vi "Problem 20 - Factorial digit sum.vi"() -> ()   [LabVIEW 2021, in "Project Euler.lvlib"]
uses:
  Project Euler.lvlib
  Utilities/Named Timers/Named Timers.lvlib
  Utilities/Numeric Utilities/Numeric Utilities.lvlib
panel:
  out "Answer = sum of digits of 100!":i32
  out "100!":string
  out "Total execution time (ms)":u32
  # "Input\nInputs to the VI"
  # "Development\nControls or indicators that are useful for development or testing, but which are not outputs of the VI."
  # "Output\nOutputs of the VI"
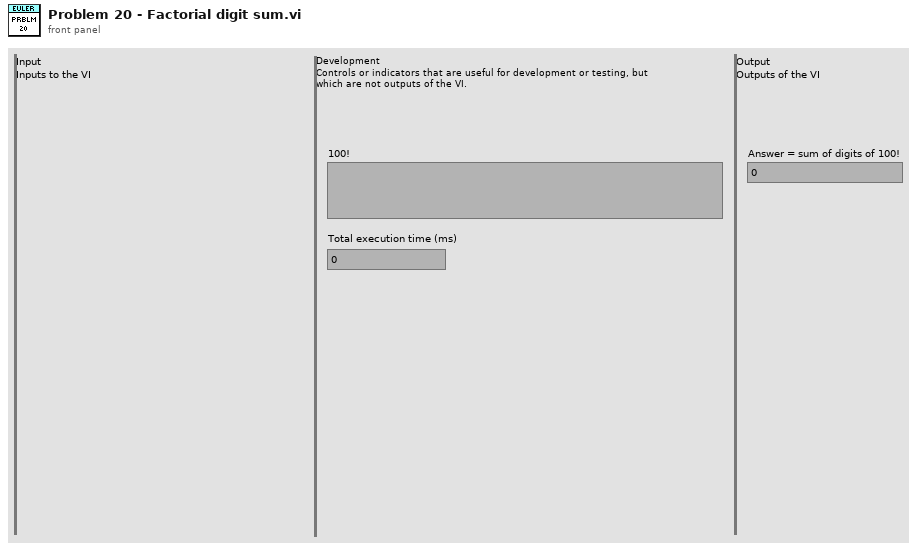
[diagram p1: front panel]
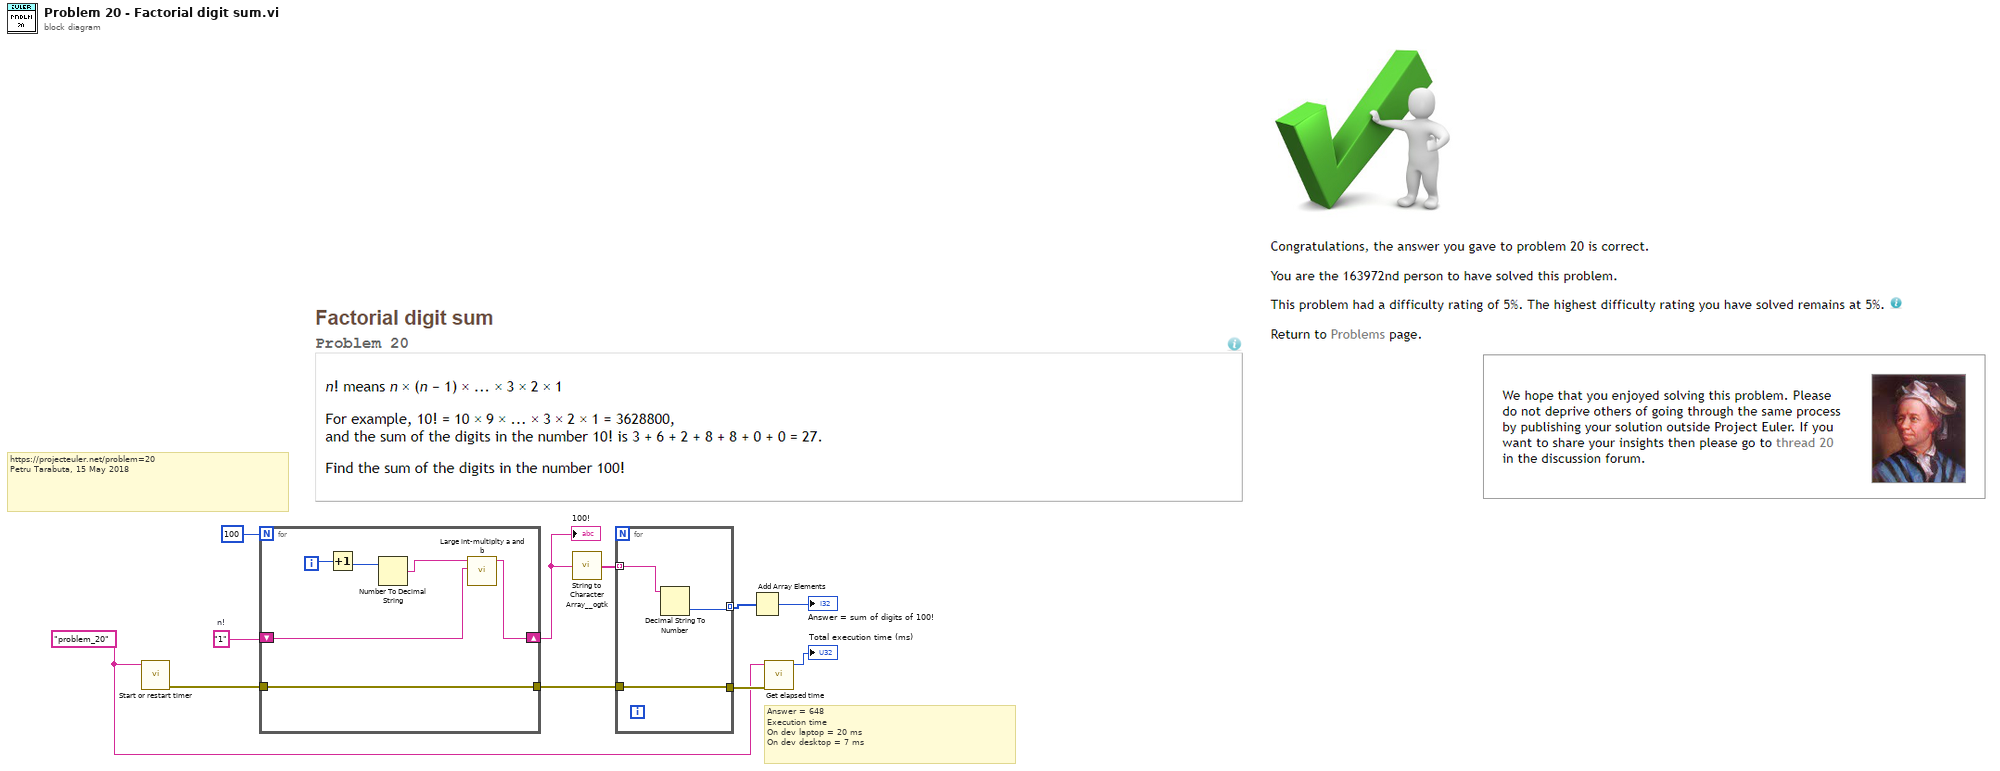
[diagram p0: block diagram]
diagram:
  w9 = "1"  # n!
  w1 = "problem_20" ("Timer name")
  # "Answer = 648\nExecution time\nOn dev laptop = 20 ms\nOn dev desktop = 7 ms"
  # "https://projecteuler.net/problem=20\nPetru Tarabuta, 15 May 2018"
  n1 = call "Start or restart timer.vi"("Timer name"=w1) -> ("error out"=w4:errorcluster)  [unwired: 10 in]
  n2 = for {
    N: 100 -> [_]
    shift-right: [w13] -> w8
    shift-left: w9 -> [w14]
    tunnel: w4 -> [w12]
    tunnel: [w12] -> w3
    i -> [w17]
    n3 = Increment(x=w17) -> (x+1=w16:i32)
    n4 = Number To Decimal String(number=w16) -> (decimal integer string=w15:string)  [unwired: 1 in]
    n5 = call "Large int-multiplty a and b.vi"("b = Large int (decimal)"=w14, "a = Large int (decimal)"=w15) -> ("c = a x b"=w13:string)  [unwired: 7 in, 2 out]
  }
  "100!" <- w8
  n6 = call <userlib>:"String to Character Array__ogtk.vi"("Input String"=w8) -> ("Character Array"=w7:string[])
  n7 = for {
    tunnel: w7 -> [w20] mode=indexing
    tunnel: [w19] -> w6 mode=indexing
    tunnel: [w18] -> w2
    tunnel: w3 -> [w18]
    n8 = Decimal String To Number(string=w20) -> (number=w19:i32)  [unwired: 2 in, 1 out]
  }
  n9 = Add Array Elements(numeric array=w6) -> (sum=→"Answer = sum of digits of 100!":i32)
  n10 = call "Get elapsed time.vi"("error in (no error)"=w2, "Timer name"=w1) -> ("Elapsed time (ms)"=→"Total execution time (ms)":u32)  [unwired: 6 in, 3 out]
